vi "AuMT8852B Test Group State.vi"(5 "EDR Tests (ON)":bool, 7 "Standard Tests (ON)":bool, 8 "error in (no error)":errorcluster, 9 "Script (3)":i32=1, 10 "Set/Get (Set)":enum16{"Set", "Get"}(ring), 11 "VISA session":refnum<visa-resource-name>) -> (0 "error out":errorcluster, 2 "error code":i32, 3 "VISA session out":refnum<visa-resource-name>, 4 "EDR Tests out":bool, 6 "Standard Tests out":bool)   [LabVIEW 2017]
doc: "Anritsu MT8852B Bluetooth Tester\n\nSelect which groups of tests are run as part of a script. The states of all the tests in the selected group are affected by this command, e.g. turning off a group will turn off all tests within that group.\n\nINPUTS\nSet/Get - whether the value is being sent to or retrieved from the instrument.\nScript - the script to access\nStandard Tests - control the state of the standard test group\nEDR Tests - control the state of the EDR test group\n\nOUTPUTS\nStandard Tests out - the current state of the standard test group.\nEDR Tests out - the current state of the EDR test group."
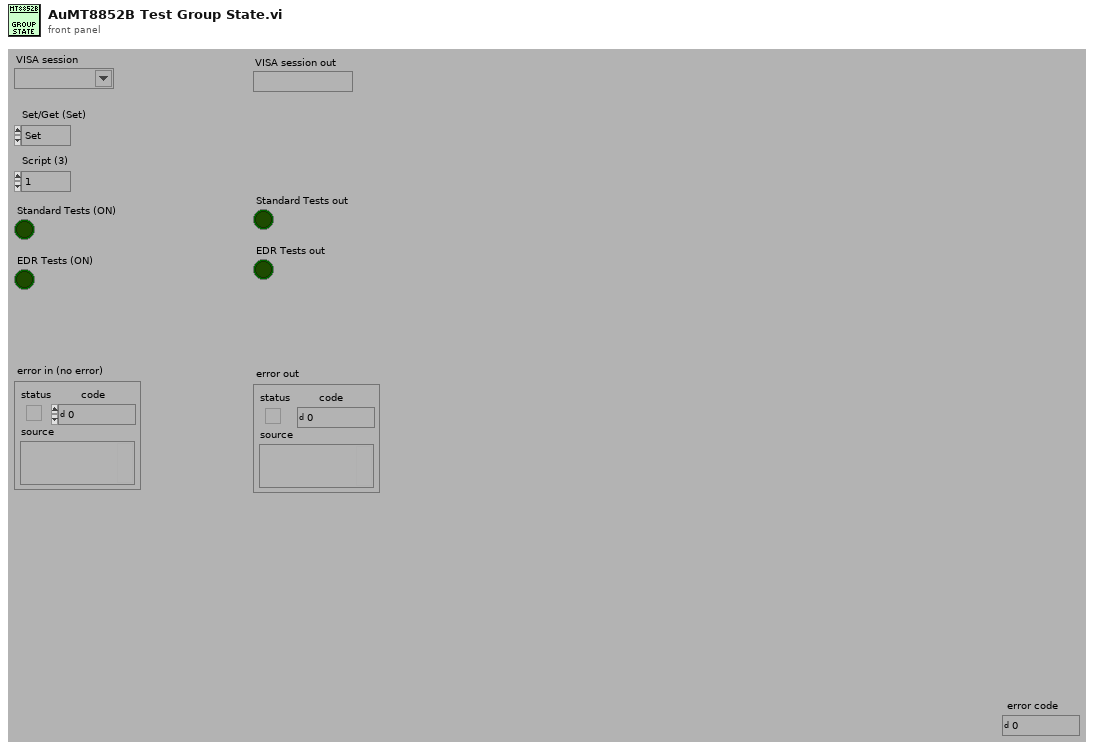
[diagram p1: front panel]
types:
  T1 = enum16{"Simulate", "Range check", "Cache", "Query instrument status"}
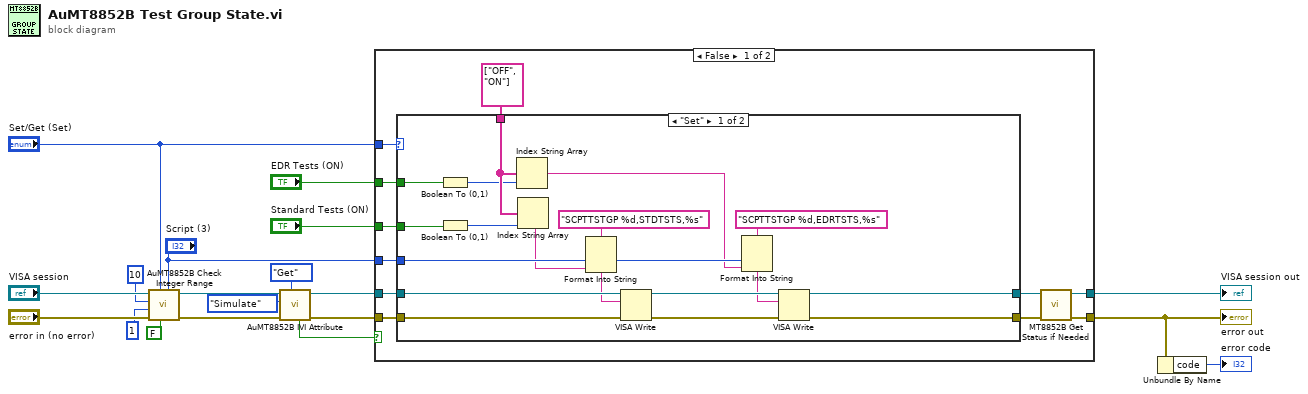
[diagram p0: block diagram]
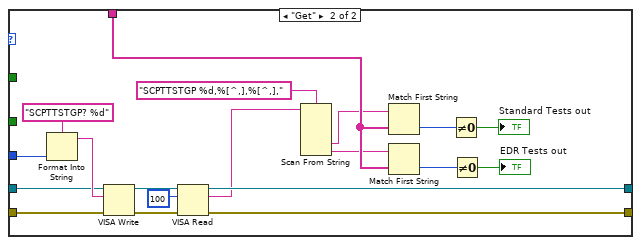
[diagram p2: hidden frame]
diagram:
  n1 = call <instrlib>:"AuMT8852B Check Integer Range.vi"("Value (0)"="Script (3)", "Check IVI flag first? (T)"=FALSE, "Set/Get (Set)"="Set/Get (Set)", "error in (no error)"="error in (no error)", "Lower limit (-1)"=1, "Upper limit (1)"=10, "VISA session"="VISA session") -> ("error out"=w12:errorcluster, "VISA session out"=w15:refnum<visa-resource-name>)  [unwired: 3 in]
  n2 = call <instrlib>:"AuMT8852B IVI Attribute.vi"("Set/Get (Set)"=enum16{"Set", "Get"}."Get", "error in (no error)"=w12, "Flag (Simulate)"=T1."Simulate", "VISA session"=w15) -> ("error out"=w13:errorcluster, "VISA session out"=w14:refnum<visa-resource-name>, "Value out"=w9:bool)  [unwired: 5 in]
  n3 = case shown="False" w9 {
    tunnel: "Set/Get (Set)" -> [w30 _]
    tunnel: [w21 w68] -> w5
    tunnel: [w22 w69] -> w19
    tunnel: w14 -> [w29 w69]
    tunnel: w13 -> [w28 w68]
    tunnel: "Script (3)" -> [w27 _]
    tunnel: "Standard Tests (ON)" -> [w25 _]
    tunnel: "EDR Tests (ON)" -> [w24 _]
    frame False {
      n4 = case shown="\"Set\"" w30 {
        tunnel: [w42 w63] -> w20
        tunnel: [w41 w64] -> w23
        tunnel: w29 -> [w48 w58]
        tunnel: w28 -> [w47 w59]
        tunnel: w27 -> [w45 w61]
        tunnel: string[] ["OFF", "ON"] ("Array Constant") -> [w40 w55]
        tunnel: w25 -> [w36 _]
        tunnel: w24 -> [w33 _]
        frame "Set" {
          n5 = Boolean To (0,1)(Boolean=w33) -> (0, 1=w34:i16)
          n6 = Boolean To (0,1)(Boolean=w36) -> (0, 1=w35:i16)
          n7 = Index String Array(1:w34, 2:w40) -> (0:w37:string)  [unwired: 1 in]
          n8 = Index String Array(1:w35, 2:w40) -> (0:w38:string)  [unwired: 1 in]
          n9 = Format Into String(format string="SCPTTSTGP %d,STDTSTS,%s" ("Format String"), w45, w38) -> (resulting string=w32:string)  [unwired: 2 in, 1 out]
          n10 = VISA Write(VISA resource name=w48, write buffer=w32, error in (no error)=w47) -> (VISA resource name out=w44:refnum<visa-resource-name>, error out=w43:errorcluster)  [unwired: 1 out]
          n11 = Format Into String(format string="SCPTTSTGP %d,EDRTSTS,%s" ("Format String"), w45, w37) -> (resulting string=w31:string)  [unwired: 2 in, 1 out]
          n12 = VISA Write(VISA resource name=w44, write buffer=w31, error in (no error)=w43) -> (VISA resource name out=w41:refnum<visa-resource-name>, error out=w42:errorcluster)  [unwired: 1 out]
        }
        frame "Get" {
          n13 = Format Into String(format string="SCPTTSTGP? %d" ("Format String"), w61) -> (resulting string=w60:string)  [unwired: 2 in, 1 out]
          n14 = VISA Write(VISA resource name=w58, write buffer=w60, error in (no error)=w59) -> (VISA resource name out=w67:refnum<visa-resource-name>, error out=w65:errorcluster)  [unwired: 1 out]
          n15 = VISA Read(VISA resource name=w67, byte count=u32 100 ("byte count (0)"), error in (no error)=w65) -> (VISA resource name out=w64:refnum<visa-resource-name>, read buffer=w57:string, error out=w63:errorcluster)  [unwired: 1 out]
          n16 = Scan From String(format string="SCPTTSTGP %d,%[^,],%[^,],", input string=w57) -> (output 2=w54:string, output 3=w53:string)  [unwired: 6 in, 3 out]
          n17 = Match First String(2:w55, 3:w54) -> (0:w52:i32)  [unwired: 1 out]
          n18 = Match First String(2:w55, 3:w53) -> (0:w51:i32)  [unwired: 1 out]
          n19 = Not Equal To 0?(x=w52) -> (x != 0?=→"Standard Tests out":bool)
          n20 = Not Equal To 0?(x=w51) -> (x != 0?=→"EDR Tests out":bool)
        }
      }
      n21 = call <instrlib>:"MT8852B Get Status if Needed.vi"("error in (no error)"=w20, "VISA session"=w23) -> ("error out"=w21:errorcluster, "VISA session out"=w22:refnum<visa-resource-name>)  [unwired: 8 in]
    }
    frame True {
    }
  }
  "error out" <- w5
  "VISA session out" <- w19
  n22 = Unbundle By Name(w5) -> ("code"=→"error code":i32)
